vi "GV_PlotRindBox.vi"(7 "type":enum16{"background", "foreground"}(ring), 9 "Vertical":i16, 10 "color(black)":u32(colorbox), 11 "Picture IN":picture) -> (3 "Picture OUT":picture)   [LabVIEW 2020, in "Sgraph_lib_V1.lvlib" / "Gviewer.lvclass"]
uses:
  Gviewer.lvclass
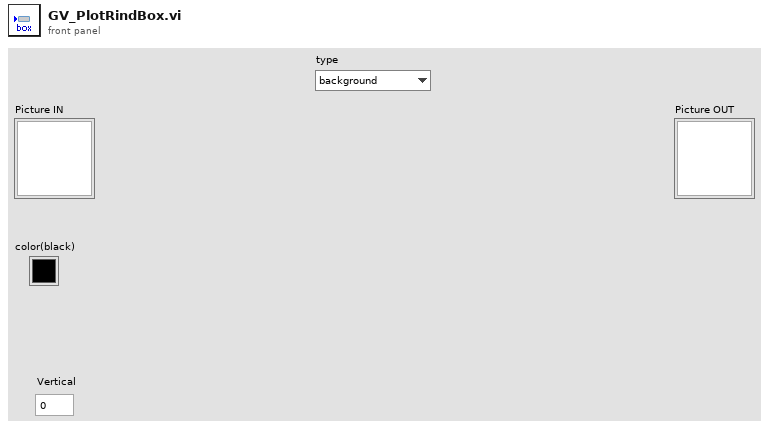
[diagram p1: front panel]
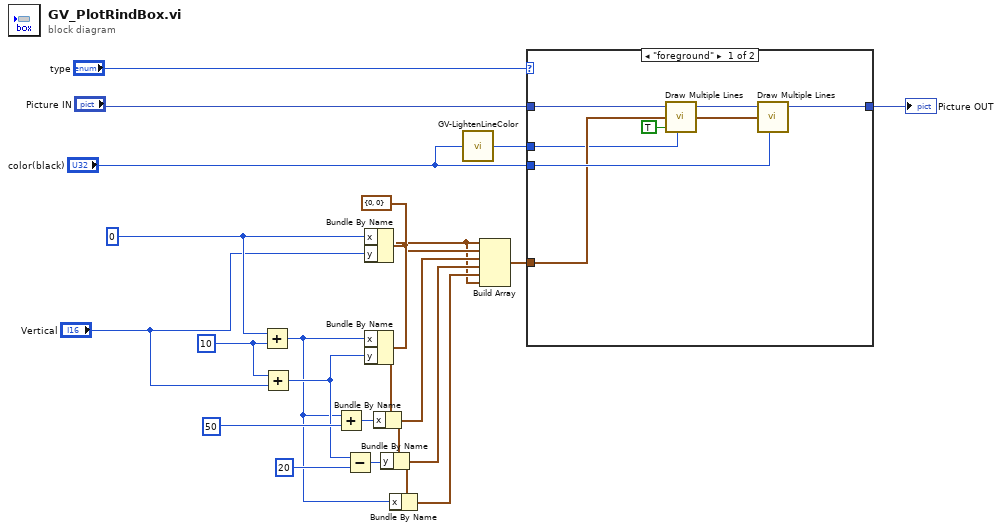
[diagram p0: block diagram]
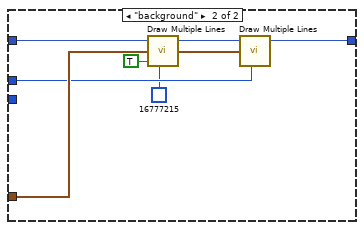
[diagram p2: hidden frame]
diagram:
  w19 = i16 10 ("y")
  w20 = i16 0 ("x")
  w17 = cluster{"x":i16, "y":i16} {"x"=0, "y"=0}
  n1 = Add(x=w20, y=w19) -> (x+y=w11:i16)
  n2 = Add(x=w19, y="Vertical") -> (x+y=w14:i16)
  n3 = Add(x=w11, y=i16 50) -> (x+y=w15:i16)
  n4 = Subtract(x=w14, y=i16 20) -> (x-y=w13:i16)
  n5 = Bundle By Name(cluster=w17, "x"=w20, "y"="Vertical") -> (w6:cluster{"x":i16, "y":i16})
  n6 = Bundle By Name(cluster=w17, "x"=w11, "y"=w14) -> (w10:cluster{"x":i16, "y":i16})
  n7 = Bundle By Name(cluster=w10, "x"=w15) -> (w9:cluster{"x":i16, "y":i16})
  n8 = Bundle By Name(cluster=w9, "y"=w13) -> (w8:cluster{"x":i16, "y":i16})
  n9 = Bundle By Name(cluster=w8, "x"=w11) -> (w7:cluster{"x":i16, "y":i16})
  n10 = call "GV-LightenLineColor.vi"("Line color"="color(black)") -> ("Light color"=w1:u32)  [unwired: 6 in]
  n11 = Build Array(w6, w10, w9, w8, w7, w6) -> (w4:cluster{"x":i16, "y":i16}[])
  n12 = case shown="\"foreground\"" "type" {
    tunnel: "Picture IN" -> [w28 w35]
    tunnel: [w26 w33] -> w5
    tunnel: "color(black)" -> [w25 _]
    tunnel: w4 -> [w23 w31]
    tunnel: w1 -> [w22 w30]
    frame "foreground" {
      n13 = call <vilib>:"Draw Multiple Lines.vi"("picture"=w28, "line endpoints"=w23, "fill?(F)"=TRUE, "color(black)"=w22) -> ("new picture"=w27:picture)  [unwired: 5 in]
      n14 = call <vilib>:"Draw Multiple Lines.vi"("picture"=w27, "line endpoints"=w23, "color(black)"=w25) -> ("new picture"=w26:picture)  [unwired: 6 in]
    }
    frame "background" {
      n15 = call <vilib>:"Draw Multiple Lines.vi"("picture"=w35, "line endpoints"=w31, "fill?(F)"=TRUE, "color(black)"=u32 16777215) -> ("new picture"=w34:picture)  [unwired: 5 in]
      n16 = call <vilib>:"Draw Multiple Lines.vi"("picture"=w34, "line endpoints"=w31, "color(black)"=w30) -> ("new picture"=w33:picture)  [unwired: 6 in]
    }
  }
  "Picture OUT" <- w5
